vi "TCP.IP Server for Ripple Detection_maybe4.vi"() -> ()   [LabVIEW 2021]
doc: "Demonstrates how to set up a basic TCP connection, send data to the specified port once a connection has been established, and terminate the connection once the data has been sent. This VI is designed to stop if the TCP connection is terminated. The data sent in this example is an array of random numbers."
panel:
  in  "Number of row to read \nat a time":i32=10000
  in  "File Path":path
  out "Iteration terminal":i32
  in  "Stop 2":bool
  in  "Client Closed":string="The client VI closed the connection."
  in  "Stop":bool
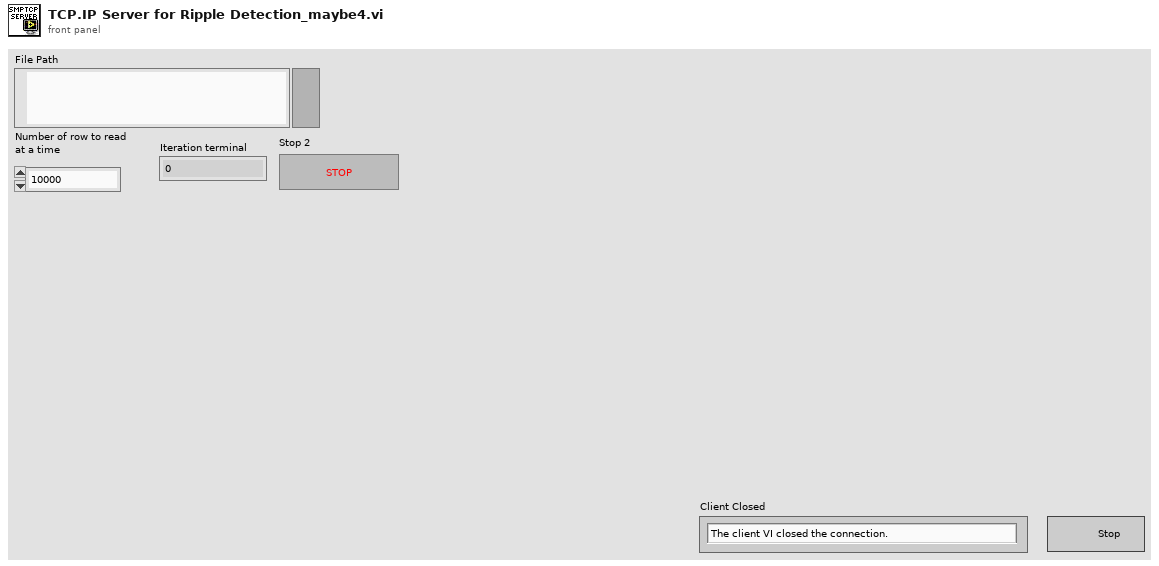
[diagram p1: front panel]
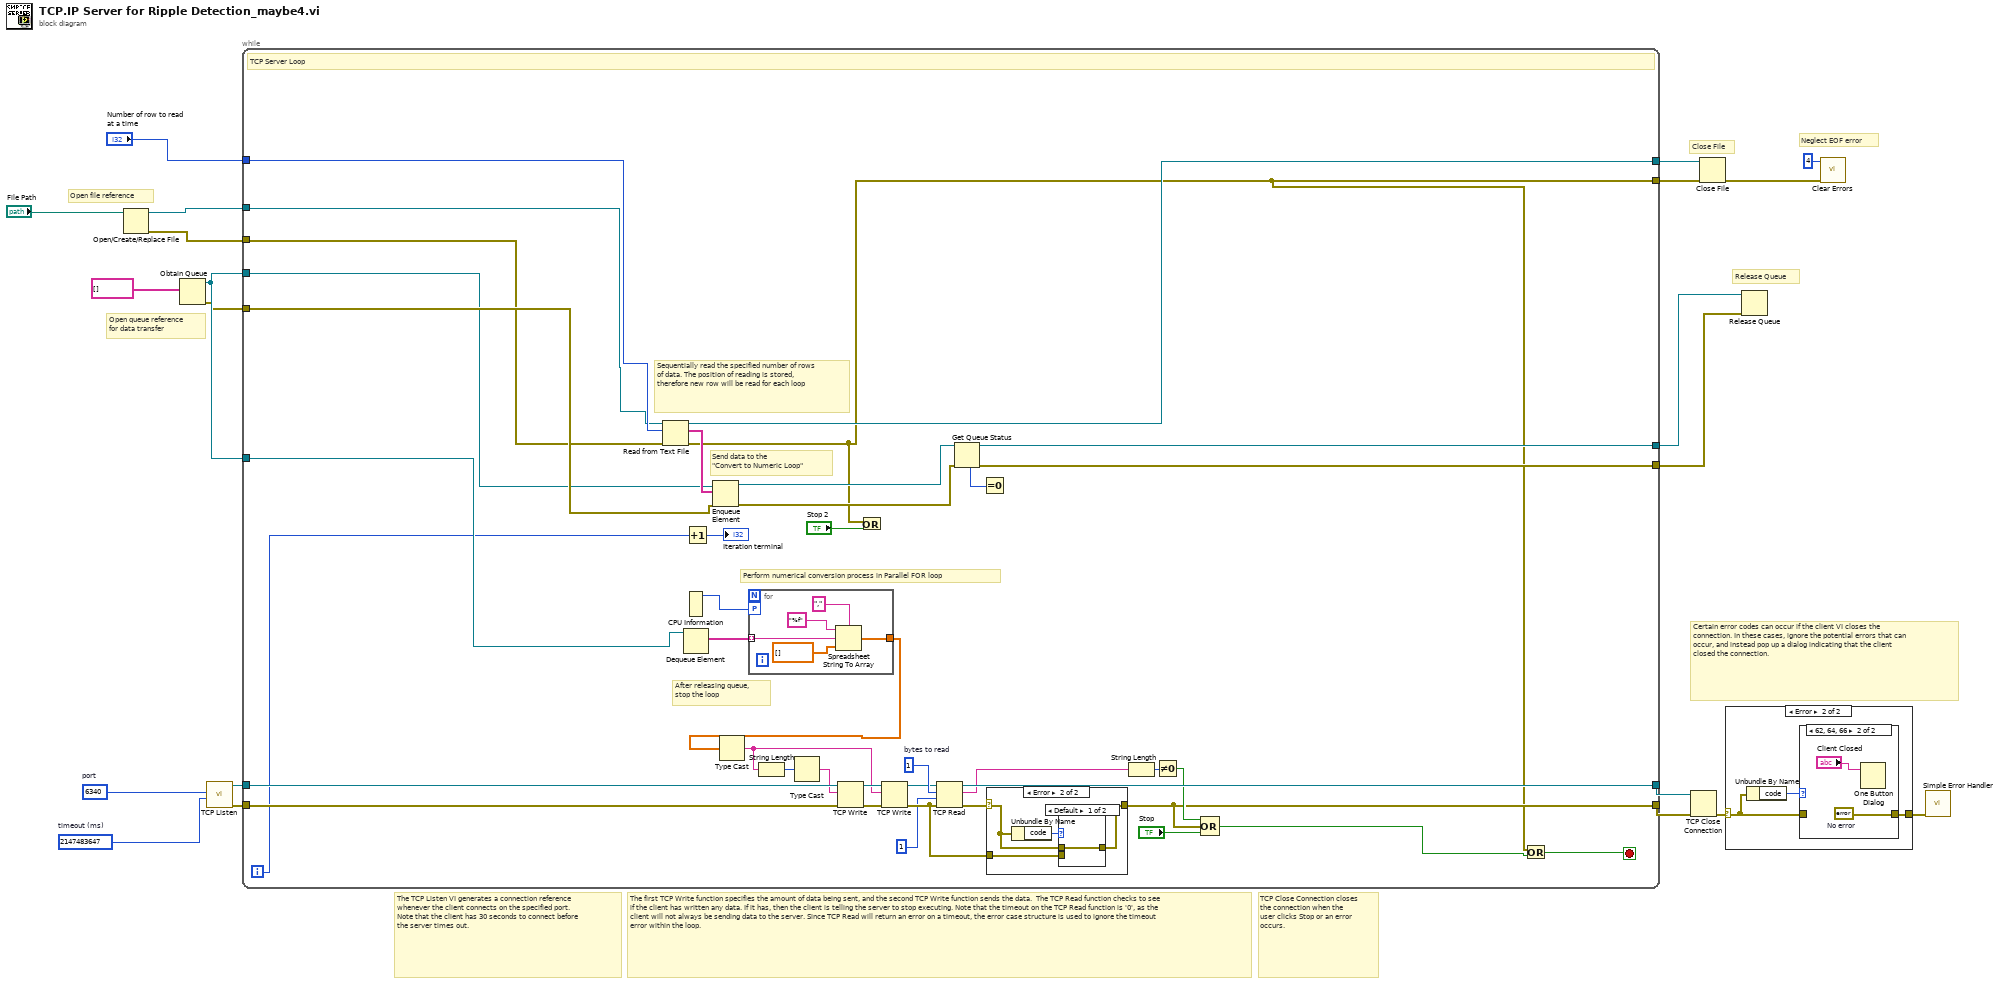
[diagram p0: block diagram]
diagram:
  w14 = u16 6340  # port
  w15 = 2147483647  # timeout (ms)
  # "Neglect EOF error"
  # "Close File"
  # "Open queue reference\nfor data transfer"
  # "Release Queue"
  # "Open file reference"
  # "TCP Close Connection closes the connection when the user clicks Stop or an error occurs."
  # "The TCP Listen VI generates a connection reference whenever the client connects on the specified port. Note that the client has 30 seconds to connect before the server times out."
  # "Certain error codes can occur if the client VI closes the connection. In these cases, ignore the potential errors that can occur, and instead pop up a dialog indicating that the client closed the connection."
  # "The first TCP Write function specifies the amount of data being sent, and the second TCP Write function sends the data.  The TCP Read function checks to see if the client has written any data. If it has, then the client is telling the server to stop executing. Note that the timeout on the TCP Read function is '0', as the client will not always be sending data to the server. Since TCP Read will return an error on a timeout, the error case structure is used to ignore the timeout error within the loop."
  n1 = Open/Create/Replace File(file path (use dialog)="File Path") -> (refnum out=w11:refnum<file>, error out=w12:errorcluster)  [unwired: 5 in, 1 out]
  n2 = Obtain Queue(element data type=string[] [] ("形式文字列")) -> (queue out=w9:refnum<queue>, error out=w8:errorcluster)  [unwired: 4 in, 1 out]
  n3 = call <vilib>:"TCP Listen.vi"("timeout ms (wait forever: -1)"=w15, "port"=w14) -> ("error out"=w16:errorcluster, "connection ID"=w17:refnum<k5>)  [unwired: 5 in, 3 out]
  n4 = while {
    tunnel: [w46] -> w20
    tunnel: [w51] -> w21
    tunnel: w17 -> [w61]
    tunnel: w16 -> [w55]
    tunnel: w11 -> [w33]
    tunnel: w12 -> [w32]
    tunnel: w9 -> [w42]
    tunnel: w9 -> [w31]
    tunnel: w8 -> [w36]
    tunnel: "Number of row to read \nat a time" -> [w34]
    tunnel: [w29] -> w6
    tunnel: [w28] -> w5
    tunnel: [w24] -> w3
    tunnel: [w25] -> w2
    i -> [w35]
    stop <- w23 stop-if-true
    w53 = 1  # bytes to read
    # "Send data to the \n\"Convert to Numeric Loop\""
    # "Sequentially read the specified number of rows of data. The position of reading is stored, therefore new row will be read for each loop"
    # "After releasing queue,\nstop the loop"
    # "Perform numerical conversion process in Parallel FOR loop"
    # "TCP Server Loop"
    n5 = Read from Text File(file (use dialog)=w33, count=w34, error in=w32) -> (refnum out=w25:refnum<file>, text=w39:string[], error out=w24:errorcluster)  [unwired: 1 in, 1 out]
    n6 = CPU Information() -> (4:w44:i32)  [unwired: 3 out]
    n7 = Dequeue Element(queue=w42) -> (element=w43:string[])  [unwired: 2 in, 3 out]
    n8 = Increment(x=w35) -> (x+1=→"Iteration terminal":i32)
    n9 = Enqueue Element(queue=w31, element=w39, error in (no error)=w36) -> (queue out=w30:refnum<queue>, error out=w27:errorcluster)  [unwired: 1 in, 1 out]
    n10 = for "Forループ" {
      tunnel: w43 -> [w63] mode=indexing
      tunnel: [w64] -> w41
      workers-P: w44 -> [_]
      n11 = Spreadsheet String To Array(delimiter (Tab)="," ("デリミタ（タブ）"), format string="%f" ("形式文字列"), spreadsheet string=w63, array type (2D Dbl)=dbl[] []) -> (array=w64:dbl[])
    }
    n12 = Type Cast(x=w41) -> (*(type *) &x=w56:string)  [unwired: 1 out]
    n13 = String Length(string=w56) -> (length=w58:i32)
    n14 = Type Cast(x=w58) -> (*(type *) &x=w57:string)  [unwired: 1 out]
    n15 = TCP Write(connection ID=w61, data in=w57, error in (no error)=w55) -> (connection ID out=w60:refnum<k5>, error out=w59:errorcluster)  [unwired: 2 out]
    n16 = Or(x=w24, y="Stop 2") -> ()  [unwired: 1 out]
    n17 = TCP Write(connection ID=w60, data in=w56, error in (no error)=w59) -> (connection ID out=w52:refnum<k5>, error out=w45:errorcluster)  [unwired: 2 out]
    n18 = TCP Read(connection ID=w52, bytes to read=w53, error in (no error)=w45, 9:1 ("timeout ms (25000)")) -> (connection ID out=w51:refnum<k5>, data out=w49:string, error out=w47:errorcluster)  [unwired: 1 out]
    n19 = Get Queue Status(queue=w30, error in (no error)=w27) -> (queue out=w29:refnum<queue>, error out=w28:errorcluster, # elements in queue=w37:i32)  [unwired: 1 in, 5 out]
    n20 = Equal To 0?(x=w37) -> ()  [unwired: 1 out]
    n21 = case shown="Error" w47 {
      selector: w47 -> [w67 w70]
      tunnel: [w67 w68] -> w46
      tunnel: w45 -> [_ w69]
      frame No Error {
      }
      frame Error {
        n22 = Unbundle By Name(w70) -> ("code"=w71:i32)
        n23 = case shown="Default" w71 {
          tunnel: w70 -> [w72 _]
          tunnel: w69 -> [_ w73]
          tunnel: [w72 w73] -> w68
          frame Default {
          }
          frame 56 {
          }
        }
      }
    }
    n24 = String Length(string=w49) -> (length=w50:i32)
    n25 = Not Equal To 0?(x=w50) -> (x != 0?=w48:bool)
    n26 = Compound Arithmetic op=OR(w48, w46, "Stop") -> (w26:bool)
    n27 = Or(x=w24, y=w26) -> (x .or. y?=w23:bool)
  }
  n28 = TCP Close Connection(connection ID=w21, error in (no error)=w20) -> (error out=w19:errorcluster)  [unwired: 2 out]
  n29 = Close File(refnum=w2, error in=w3) -> (error out=w4:errorcluster)  [unwired: 1 out]
  n30 = case shown="Error" w19 {
    selector: w19 -> [w74 w76]
    tunnel: [w74 w75] -> w18
    frame No Error {
    }
    frame Error {
      n31 = Unbundle By Name(w76) -> ("code"=w77:i32)
      n32 = case shown="62, 64, 66" w77 {
        tunnel: w76 -> [w78 _]
        tunnel: [w78 w80] -> w75
        frame Default {
        }
        frame 62, 64, 66 {
          w80 = errorcluster {"status"=FALSE, "code"=0, "source"=""}  # No error
          n33 = One Button Dialog(message="Client Closed") -> ()  [unwired: 1 in, 1 out]
        }
      }
    }
  }
  n34 = Release Queue(queue=w6, error in (no error)=w5) -> ()  [unwired: 1 in, 3 out]
  n35 = call <vilib>:"Clear Errors.vi"("error in (no error)"=w4, "specific error code to clear (0: all)"=4) -> ()  [unwired: 4 in, 2 out]
  n36 = call <vilib>:"Simple Error Handler.vi"("error in (no error)"=w18) -> ()  [unwired: 1 in, 8 out]
